vi "Configure Session.vi"(8 "error in":errorcluster, 11 "Plugin in":refnum<class "PXIe4113 DUT Power Control Replacement.lvclass">) -> (0 "error out":errorcluster, 3 "Plugin out":refnum<class "PXIe4113 DUT Power Control Replacement.lvclass">)   [LabVIEW 2026, in "PXIe4113 DUT Power Control Replacement.lvlib" / "PXIe4113 DUT Power Control Replacement.lvclass"]
uses:
  PXIe4113 DUT Power Control Replacement.lvclass
  C:/Program Files/National Instruments/LabVIEW 2026/vi.lib/FlexLogger/SDK/PluginSDK.lvlibp/PEFClasses/SDK/Plugin/Plugin.lvclass
  PXIe4113 DUT Power Control Replacement.lvclass/PXIe4113 DUT Power Control Replacement.ctl
  <vilib>/FlexLogger/SDK/PluginSDK.lvlibp/PEFClasses/SDK/Plugin/ParameterAccess/Read String.vi
  <vilib>/FlexLogger/SDK/PluginSDK.lvlibp/PEFClasses/SDK/Plugin/Plugin.lvclass
  C:/Program Files/National Instruments/LabVIEW 2026/vi.lib/FlexLogger/SDK/PluginSDK.lvlibp/PEFClasses/SDK/Processing Element/Processing Element.lvclass
  C:/Users/localadmin/Documents/LabVIEW Projects/FlexLogger IO Plug-ins/PXIe4113 DUT Power Control Replacement/PXIe4113 DUT Power Control Replacement.lvclass
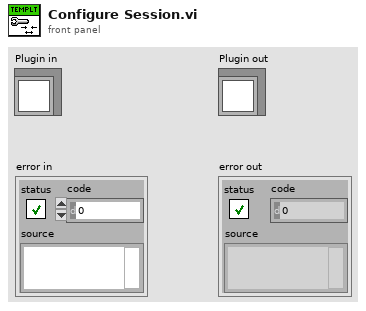
[diagram p1: front panel]
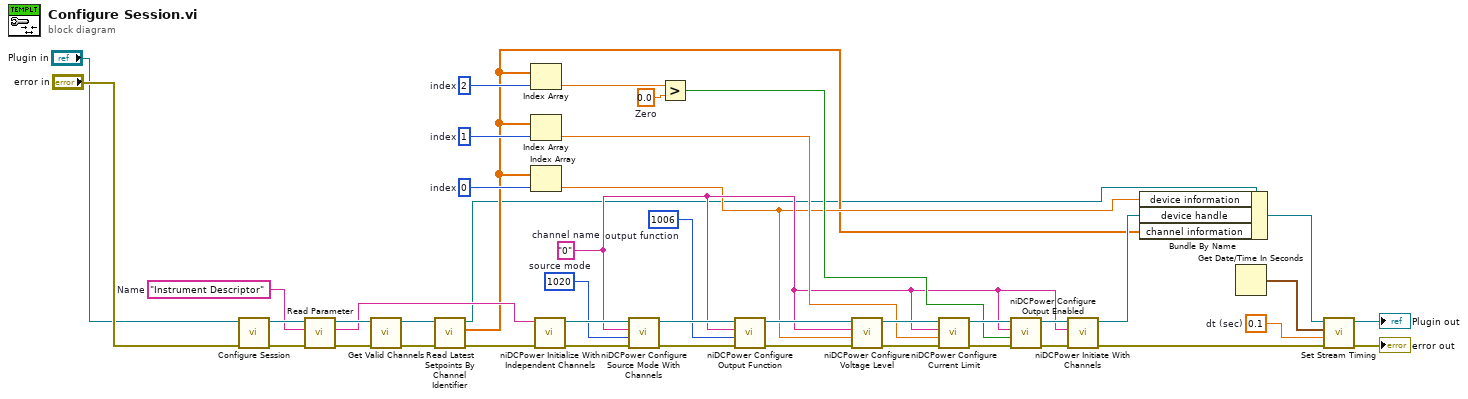
[diagram p0: block diagram]
diagram:
  w4 = 0.1  # dt (sec)
  w17 = 0.0  # Zero
  w25 = 1006  # output function
  w28 = 1020  # source mode
  w12 = "0"  # channel name
  w32 = 2  # index
  w33 = 1  # index
  w34 = 0  # index
  w40 = "Instrument Descriptor"  # Name
  n1 = call-parent "Configure Session.vi"("error in (no error)"="error in", "Processing Element in"="Plugin in") -> ("error out"=w39:errorcluster, "Processing Element out"=w41:refnum<class "PXIe4113 DUT Power Control Replacement.lvclass">)  [unwired: 8 in]
  n2 = call-poly <vilib>:"Read Parameter.vi"("error in (no error)"=w39, "Name"=w40, "Plugin in"=w41) -> ("error out"=w37:errorcluster, "Value"=w31:string, "Plugin out"=w38:refnum<class "PXIe4113 DUT Power Control Replacement.lvclass">)  [unwired: 5 in, 1 out]
  n3 = call <vilib>:"Get Valid Channels.vi"("error in (no error)"=w37, "Plugin in"=w38) -> ("error out"=w35:errorcluster, "Plugin out"=w36:refnum<class "PXIe4113 DUT Power Control Replacement.lvclass">)  [unwired: 7 in, 1 out]
  n4 = call <vilib>:"Read Latest Setpoints By Channel Identifier.vi"("error in (no error)"=w35, "Plugin in"=w36) -> ("error out"=w30:errorcluster, "Channel Setpoints"=w8:dbl[], "Plugin out"=w7:refnum<class "PXIe4113 DUT Power Control Replacement.lvclass">)  [unwired: 6 in, 1 out]
  n5 = Index Array(array=w8, index=w32) -> (element=w18:dbl)
  n6 = Index Array(array=w8, index=w33) -> (element=w20:dbl)
  n7 = Index Array(array=w8, index=w34) -> (element=w10:dbl)
  n8 = call <instrlib>:"niDCPower Initialize With Independent Channels.vi"("error in (no error)"=w30, "resource name"=w31) -> ("error out"=w27:errorcluster, "instrument handle out"=w29:refnum<k15>)  [unwired: 8 in]
  n9 = call <instrlib>:"niDCPower Configure Source Mode With Channels.vi"("error in (no error)"=w27, "source mode"=w28, "channel name"=w12, "instrument handle"=w29) -> ("error out"=w24:errorcluster, "instrument handle out"=w26:refnum<k15>)  [unwired: 6 in]
  n10 = Greater?(x=w18, y=w17) -> (0:w15:bool)
  n11 = call <instrlib>:"niDCPower Configure Output Function.vi"("error in (no error)"=w24, "output function"=w25, "channel name"=w12, "instrument handle"=w26) -> ("error out"=w22:errorcluster, "instrument handle out"=w23:refnum<k15>)  [unwired: 6 in]
  n12 = call <instrlib>:"niDCPower Configure Voltage Level.vi"("error in (no error)"=w22, "voltage level"=w10, "channel name"=w12, "instrument handle"=w23) -> ("error out"=w19:errorcluster, "instrument handle out"=w21:refnum<k15>)  [unwired: 6 in]
  n13 = call <instrlib>:"niDCPower Configure Current Limit.vi"("error in (no error)"=w19, "current limit"=w20, "channel name"=w12, "instrument handle"=w21) -> ("error out"=w14:errorcluster, "instrument handle out"=w16:refnum<k15>)  [unwired: 6 in]
  n14 = call <instrlib>:"niDCPower Configure Output Enabled.vi"("error in (no error)"=w14, "output enabled"=w15, "channel name"=w12, "instrument handle"=w16) -> ("error out"=w11:errorcluster, "instrument handle out"=w13:refnum<k15>)  [unwired: 6 in]
  n15 = call <instrlib>:"niDCPower Initiate With Channels.vi"("error in (no error)"=w11, "channel name"=w12, "instrument handle"=w13) -> ("error out"=w3:errorcluster, "instrument handle out"=w9:refnum<k15>)  [unwired: 7 in]
  n16 = Bundle By Name(cluster=w7, "device information"=w10, "device handle"=w9, "channel information"=w8) -> (w6:refnum<class "PXIe4113 DUT Power Control Replacement.lvclass">)
  n17 = Get Date/Time In Seconds() -> (seconds since 1Jan1904=w5:timestamp)
  n18 = call-dynamic "Set Stream Timing.vi"("error in (no error)"=w3, "dt(sec)"=w4, "Start Time"=w5, "Plugin in"=w6) -> ("error out"=→"error out":errorcluster, "Plugin out"=→"Plugin out":refnum<class "PXIe4113 DUT Power Control Replacement.lvclass">)  [unwired: 6 in]
